vi "TCU Tags.vi"(11 "TCU Module Configs":T1[](array[typedef]) {"Settings"."Julabo FP-50 Settings"."Pump Power" min=0 max=8 step=1; "Settings"."Lauda Settings"."Pump Power" min=0 max=8 step=1}) -> (1 "TCU Module Tags":T9, 2 "TCU Module Tags Array":T9[](array[typedef]), 3 "All Boolean Tags 5":string[](array[string]), 4 "All  Numeric Tags 5":string[](array[string]))   [LabVIEW 2018]
uses:
  TCU Module/TCU Module Folder/TCU Module Tag Names Cluster.ctl
  TCU Module/TCU Module Folder/TCU Module Config Cluster.ctl
  <vilib>/Utility/miscctls.llb/LVPoint32TypeDef.ctl
  TCU Module/TCU Module Folder/TCU Module Settings Cluster.ctl
  TCU Module/TCU Module Folder/Measure Instrument/Output Devices.ctl
  Huber TCU/Huber Settings.ctl
  Lauda Integral XT-150 TCU/Lauda Settings.ctl
  Julabo Type 1 TCU/Julabo Type 1 TCU Folder/Julabo FP-50 Settings.ctl
  Huber Unistat 410 TCU/Huber Unistat 410 Settings.ctl
  TCU Module/TCU Module Folder/TCU Module.lvlib
  Huber TCU/Huber Ministat 230 TCU.lvlib
  Lauda Integral XT-150 TCU/Lauda TCU.lvlib
  Julabo Type 1 TCU/Julabo Type 1 TCU Folder/Julabo Type FP-50 TCU.lvlib
  Huber Unistat 410 TCU/Huber Unistat 410 TCU.lvlib
panel:
  # "Output Instruments"
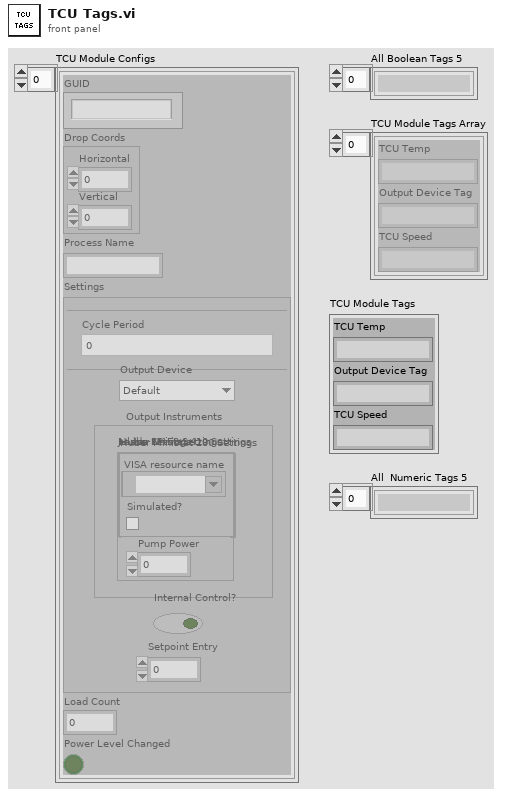
[diagram p1: front panel]
types:
  T1 = typedef "TCU Module.lvlib/TCU Module Config Cluster.ctl" = cluster{"GUID":string, "Drop Coords":T2, "Process Name":string, "Settings":T3, "Load Count":i32, "Power Level Changed":bool}
  T2 = typedef "LVPoint32TypeDef.ctl" = cluster{"Horizontal":i32, "Vertical":i32}
  T3 = typedef "TCU Module.lvlib/TCU Module Settings Cluster.ctl" = cluster{"Cycle Period":dbl, "Setpoint Entry":dbl, "Output Device":T4, "Huber Ministat 230 Settings":T5, "Lauda Settings":T6, "Julabo FP-50 Settings":T7, "Internal Control?":bool, "Huber Unistat 410 Settings":T8}
  T4 = typedef "Output Devices.ctl" = enum16{"Default", "Huber Ministat 230", "Huber Unistat 410", "Lauda XT-150", "Julabo FP-50"}
  T5 = typedef "Huber Ministat 230 TCU.lvlib/Huber Settings.ctl" = cluster{"VISA resource name":refnum<visa-resource-name>, "Simulated?":bool}
  T6 = typedef "Lauda TCU.lvlib/Lauda Settings.ctl" = cluster{"VISA resource name":refnum<visa-resource-name>, "Simulated?":bool, "Pump Power":i32}
  T7 = typedef "Julabo Type FP-50 TCU.lvlib/Julabo FP-50 Settings.ctl" = cluster{"VISA resource name":refnum<visa-resource-name>, "Simulated?":bool, "Pump Power":i32}
  T8 = typedef "Huber Unistat 410 TCU.lvlib/Huber Unistat 410 Settings.ctl" = cluster{"VISA resource name":refnum<visa-resource-name>, "Simulated?":bool}
  T9 = typedef "TCU Module.lvlib/TCU Module Tag Names Cluster.ctl" = cluster{"TCU Temp":string, "Output Device Tag":string, "TCU Speed":string}
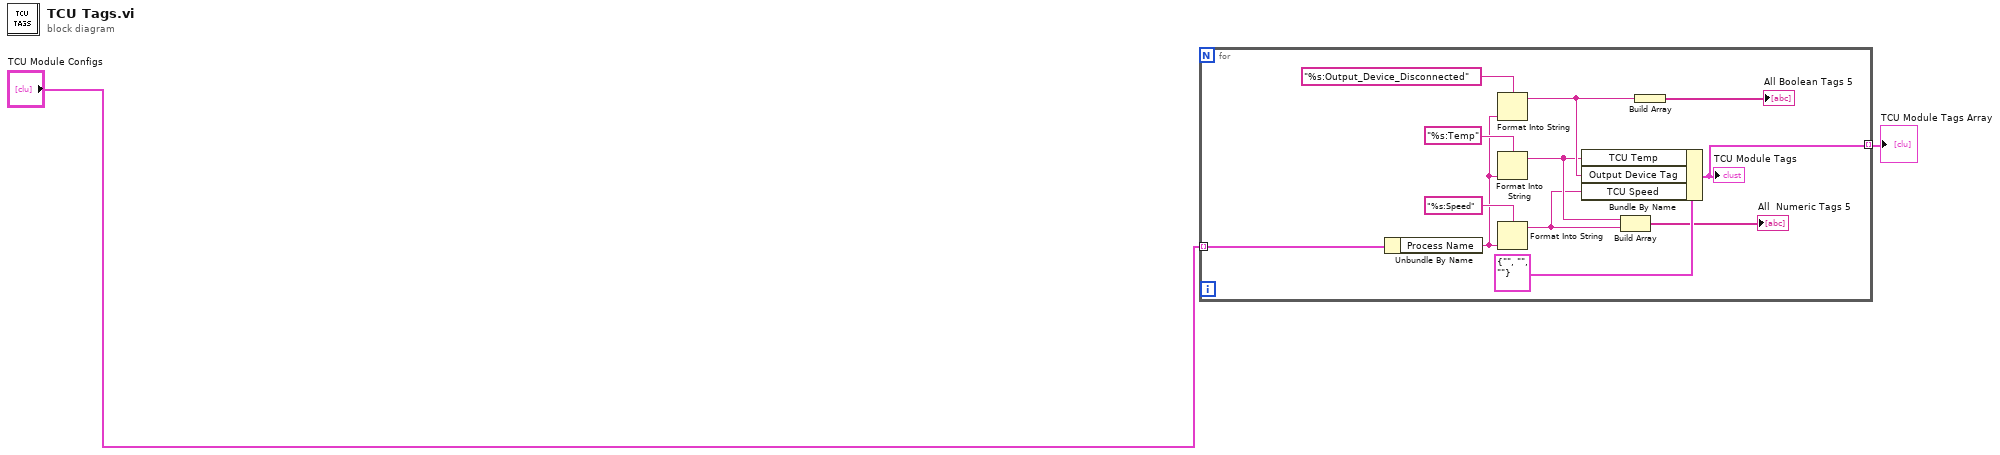
[diagram p0: block diagram]
diagram:
  n1 = for {
    tunnel: "TCU Module Configs" -> [w5] mode=indexing
    tunnel: [w3] -> w2 mode=indexing
    n2 = Unbundle By Name(w5) -> ("Process Name"=w4:string)
    n3 = Format Into String(format string="%s:Output_Device_Disconnected", w4) -> (resulting string=w14:string)  [unwired: 2 in, 1 out]
    n4 = Format Into String(format string="%s:Temp", w4) -> (resulting string=w9:string)  [unwired: 2 in, 1 out]
    n5 = Format Into String(format string="%s:Speed", w4) -> (resulting string=w6:string)  [unwired: 2 in, 1 out]
    n6 = Bundle By Name(cluster=T9 {"TCU Temp"="", "Output Device Tag"="", "TCU Speed"=""} ("Feed Module Tag Names"), "TCU Temp"=w9, "Output Device Tag"=w14, "TCU Speed"=w6) -> (w3:T9)
    "TCU Module Tags" <- w3
    n7 = Build Array(w9, w6) -> (→"All  Numeric Tags 5":string[])
    n8 = Build Array(w14) -> (→"All Boolean Tags 5":string[])
  }
  "TCU Module Tags Array" <- w2
